vi "Set Supply State.vi"(8 "error in (no error)":errorcluster, 9 "Output":bool, 10 "Supply_ID":string, 11 "Chronometer in":refnum<class "Chronometer.lvclass">) -> (0 "error out":errorcluster, 3 "Chronometer out":refnum<class "Chronometer.lvclass">)   [LabVIEW 2023, in "Chronometer.lvlib" / "Chronometer.lvclass"]
uses:
  Library/Chronometer.lvclass
  Library/Chronometer.lvclass/Chronometer.ctl
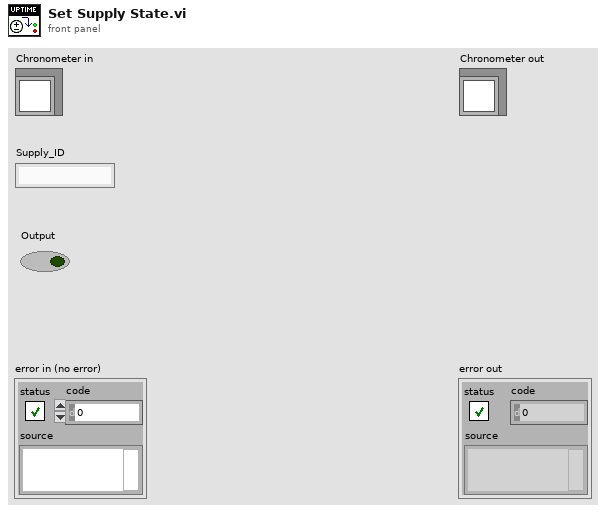
[diagram p1: front panel]
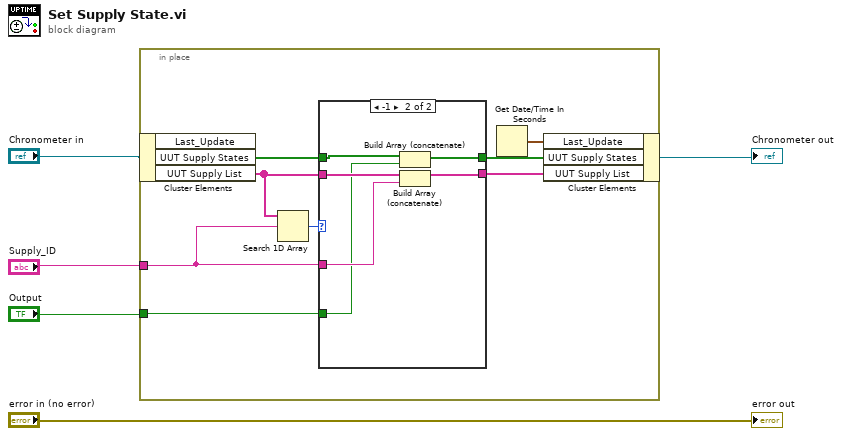
[diagram p0: block diagram]
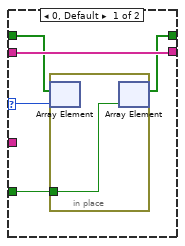
[diagram p2: hidden frame]
diagram:
  n1 = in-place {
    in-place-border: "Supply_ID" -> [w12]
    in-place-border: "Output" -> [w9]
    n2 = in-place-cluster #1("Chronometer in") -> ("UUT Supply States"=w10:bool[], "UUT Supply List"=w11:string[])  [unwired: 1 out]
    n3 = Search 1D Array(1D array=w11, element=w12) -> (index of element=w13:i32)  [unwired: 1 in]
    n4 = case shown="-1" w13 {
      selector: w13 -> [w15 _]
      tunnel: w12 -> [_ w23]
      tunnel: w11 -> [w18 w25]
      tunnel: w10 -> [w17 w24]
      tunnel: w9 -> [w14 w22]
      tunnel: [w16 w21] -> w8
      tunnel: [w18 w20] -> w7
      frame 0, Default {
        n5 = in-place {
          in-place-border: w14 -> [w19]
          n6 = in-place-array #2(w17, w15) -> ()  [unwired: 1 out]
          n7 = in-place-array #2(w19) -> (w16:bool[])  [unwired: 1 out]
        }
      }
      frame -1 {
        n8 = Build Array (concatenate)(w24, w22) -> (w21:bool[])
        n9 = Build Array (concatenate)(w25, w23) -> (w20:string[])
      }
    }
    n10 = Get Date/Time In Seconds() -> (seconds since 1Jan1904=w6:timestamp)
    n11 = in-place-cluster #1("Last_Update"=w6, "UUT Supply States"=w8, "UUT Supply List"=w7) -> (→"Chronometer out":refnum<class "Chronometer.lvclass">)
  }
  "error out" <- "error in (no error)"
